vi "Start.vi"(8 "error in (no error)":errorcluster, 11 "VISA GPS in":refnum<class "VISA GPS.lvclass">) -> (0 "error out":errorcluster, 3 "VISA GPS out":refnum<class "VISA GPS.lvclass">)   [LabVIEW 2020, in "VISA GPS.lvlib" / "VISA GPS.lvclass"]
uses:
  VISA GPS.lvclass
  VISA GPS.lvclass/VISA GPS.ctl
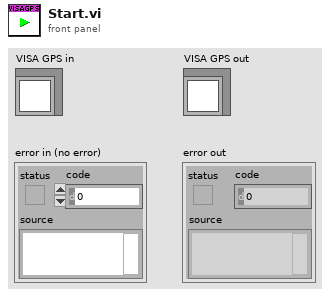
[diagram p1: front panel]
types:
  T1 = typedef "nmea.lvlib/VISA GPS.lvclass/Ref Data.ctl" = cluster{"Close":bool}
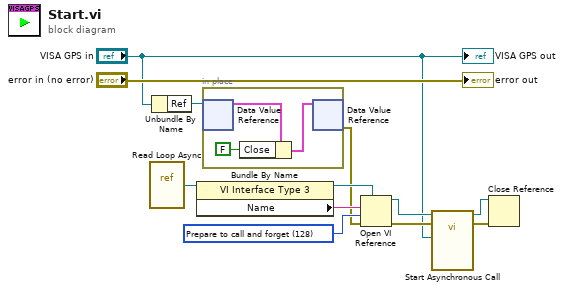
[diagram p0: block diagram]
diagram:
  w6 = 128 items=["Record modifications"=1, "Open templates for editing"=2, "Prompt user to save"=4, "Prepare for reentrant run"=8, "Prompt to find missing subVIs"=16, "Hide loading dialog box"=32, "Enable simultaneous calls"=64, "Prepare to call and forget"=128, "Simultaneous call and forget"=192, "Prepare to call and collect"=256, "Simultaneous call and collect"=320]
  n1 = vi-ref "Read Loop Async.vi"() -> (w4:refnum<vi>)
  n2 = Unbundle By Name("VISA GPS in") -> ("Ref"=w3:refnum<data-value>)
  n3 = property class="VI Interface Type 3"(reference=w4) -> (reference out=w7:refnum<vi>, "Name"=w5:string)  [unwired: 1 in, 1 out]
  n4 = in-place {
    n5 = in-place-dvr #1(w3) -> (w15:T1)  [unwired: 1 out]
    n6 = Bundle By Name(cluster=w15, "Close"=FALSE) -> (w14:T1)
    n7 = in-place-dvr #1(w14) -> (w1:errorcluster)  [unwired: 1 out]
  }
  n8 = Open VI Reference(type specifier VI Refnum (for type only)=w7, vi path=w5, options=w6, error in (no error)=w1) -> (vi reference=w9:refnum<vi>, error out=w8:errorcluster)  [unwired: 2 in]
  n9 = call-by-ref "Start Asynchronous Call"(reference=w9, error in=w8, "VISA GPS in"="VISA GPS in") -> (reference out=w11:refnum<vi>, error out=w10:errorcluster)  [unwired: 11 in]
  n10 = Close Reference(reference=w11, error in (no error)=w10) -> ()  [unwired: 1 out]
  "error out" <- "error in (no error)"
  "VISA GPS out" <- "VISA GPS in"
